vi "CalculateWaveform.vi"(8 "error out":errorcluster, 11 "Waveform Specification":T1={"X SignalType"=enum."Sine Wave", "X Offset"=2.0, "X Frequency"=100.0, "X Amplitude"=1.0, "X Phase"=0.0, "Y SignalType"=enum."Sine Wave", "Y Offset"=2.0, "Y Frequency"=100.0, "Y Amplitude"=1.0, "Y Phase"=0.0, "Z SignalType"=enum."Sine Wave", "Z Offset"=2.0, "Z Frequency"=100.0, "Z Amplitude"=1.0, "Z Phase"=0.0}) -> (0 "error in":errorcluster, 3 "Array":waveform(dbl)[](array[waveform]))   [LabVIEW 2017, in "WaveformGenerator.lvlib"]
uses:
  WaveformGenerator.lvlib
  WaveformSpecs.ctl
  <vilib>/measure/NI_MABase.lvlib
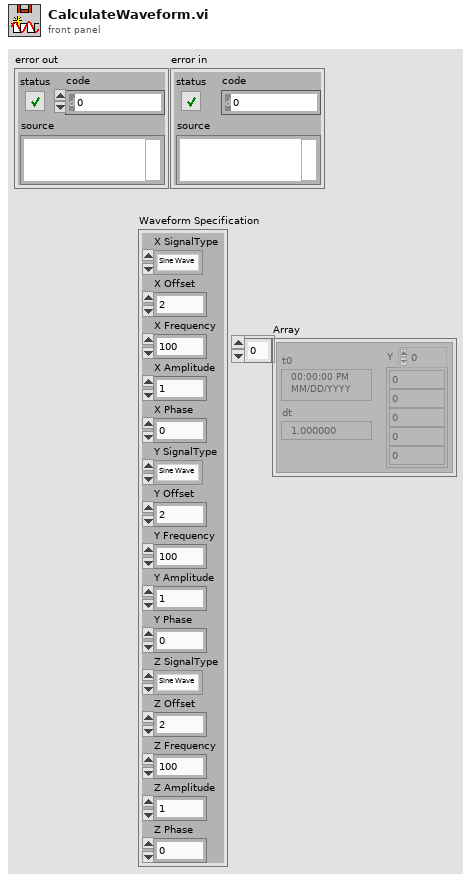
[diagram p1: front panel]
types:
  T1 = typedef "WaveformGenerator.lvlib/WaveformSpecs.ctl" = cluster{"X SignalType":enum16{"Sine Wave", "Triangle Wave", "Square Wave", "Sawtooth Wave"}, "X Offset":dbl, "X Frequency":dbl, "X Amplitude":dbl, "X Phase":dbl, "Y SignalType":enum16{"Sine Wave", "Triangle Wave", "Square Wave", "Sawtooth Wave"}, "Y Offset":dbl, "Y Frequency":dbl, "Y Amplitude":dbl, "Y Phase":dbl, "Z SignalType":enum16{"Sine Wave", "Triangle Wave", "Square Wave", "Sawtooth Wave"}, "Z Offset":dbl, "Z Frequency":dbl, "Z Amplitude":dbl, "Z Phase":dbl}
  T2 = enum16{"Sine Wave", "Triangle Wave", "Square Wave", "Sawtooth Wave"}
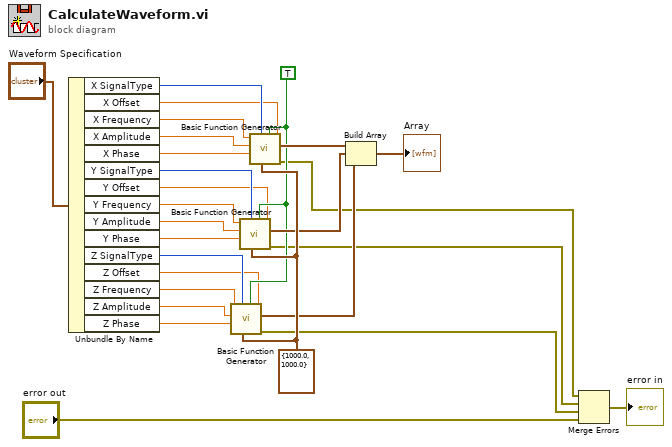
[diagram p0: block diagram]
diagram:
  w27 = cluster{"Fs":dbl, "#s":dbl} {"Fs"=1000.0, "#s"=1000.0} ("sampling info")
  w22 = TRUE ("reset signal")
  n1 = Unbundle By Name("Waveform Specification") -> ("X SignalType"=w20:T2, "X Offset"=w19:dbl, "X Frequency"=w18:dbl, "X Amplitude"=w17:dbl, "X Phase"=w16:dbl, "Y SignalType"=w15:T2, "Y Offset"=w14:dbl, "Y Frequency"=w13:dbl, "Y Amplitude"=w11:dbl, "Y Phase"=w12:dbl, "Z SignalType"=w10:T2, "Z Offset"=w9:dbl, "Z Frequency"=w6:dbl, "Z Amplitude"=w7:dbl, "Z Phase"=w8:dbl)
  n2 = call <vilib>:"Basic Function Generator.vi"("offset"=w9, "reset signal"=w22, "sampling info"=w27, "signal type"=w10, "phase"=w8, "amplitude"=w7, "frequency"=w6) -> ("error out"=w2:errorcluster, "signal out"=w23:waveform(dbl))  [unwired: 2 in, 1 out]
  n3 = call <vilib>:"Basic Function Generator.vi"("offset"=w14, "reset signal"=w22, "sampling info"=w27, "signal type"=w15, "phase"=w12, "amplitude"=w11, "frequency"=w13) -> ("error out"=w3:errorcluster, "signal out"=w24:waveform(dbl))  [unwired: 2 in, 1 out]
  n4 = call <vilib>:"Basic Function Generator.vi"("offset"=w19, "reset signal"=w22, "sampling info"=w27, "signal type"=w20, "phase"=w16, "amplitude"=w17, "frequency"=w18) -> ("error out"=w4:errorcluster, "signal out"=w25:waveform(dbl))  [unwired: 2 in, 1 out]
  n5 = Build Array(w25, w24, w23) -> (→"Array":waveform(dbl)[])
  n6 = Merge Errors(w4, w3, w2, "error out") -> (→"error in":errorcluster)
